vi "DAC Configure.vi"(8 "error in":errorcluster, 11 "DAC Vacum Pressure in":refnum<class "DAC Vacum Pressure.lvclass">) -> (0 "error out":errorcluster, 3 "DAC Vacum Pressure out":refnum<class "DAC Vacum Pressure.lvclass">)   [LabVIEW 2019, in "DAC.lvlib" / "DAC Vacum Pressure.lvclass"]
uses:
  DAC Vacum Pressure.lvclass
  C:/Users/krio/Documents/LV_Projects/test-stand/App/DAC/DAC.lvclass
  DAC.lvclass/DAC.ctl
  DAC Vacum Pressure.lvclass/DAC Vacum Pressure.ctl
  DAC.lvclass
  <vilib>/DAQmx/create/channels.llb/DAQmx Create Channel (AI-Current-Basic).vi
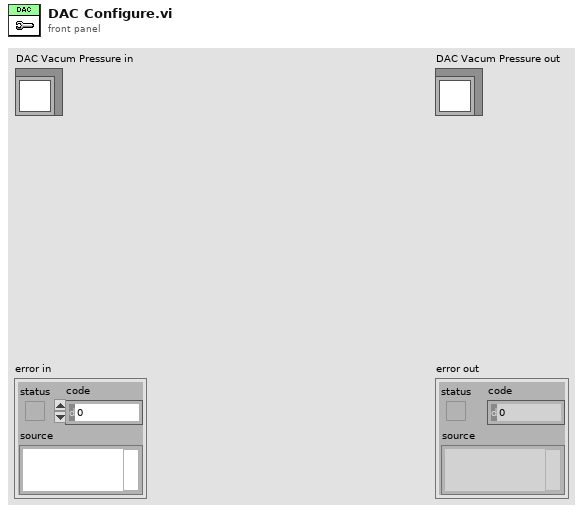
[diagram p1: front panel]
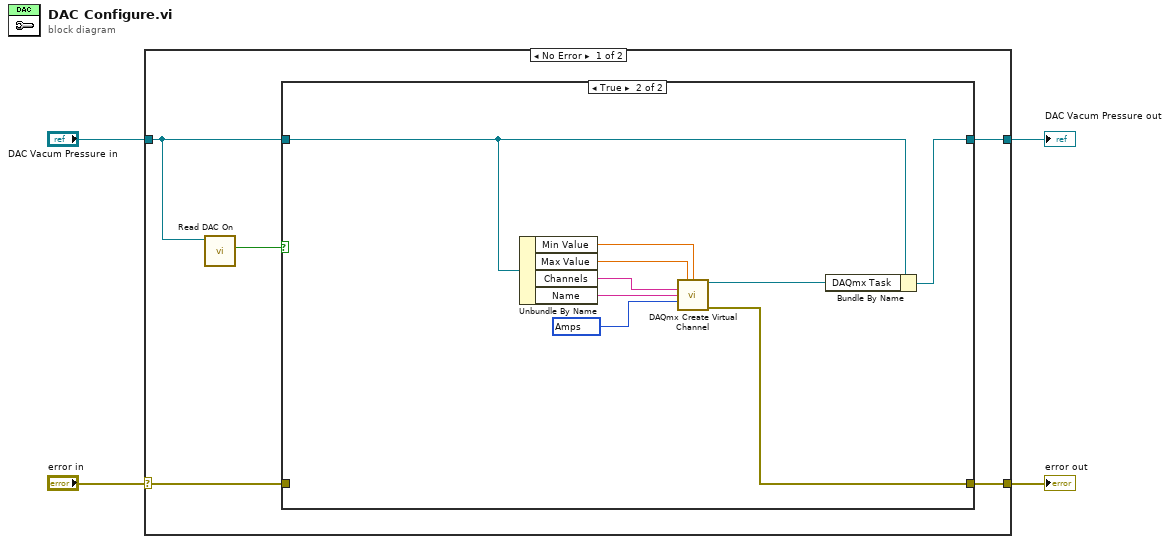
[diagram p0: block diagram]
diagram:
  n1 = case shown="No Error" "error in" {
    selector: "error in" -> [w6 w22]
    tunnel: [w5 w22] -> w4
    tunnel: [w7 w21] -> w3
    tunnel: "DAC Vacum Pressure in" -> [w9 w21]
    frame No Error {
      n2 = call "Read DAC On.vi"("DAC in"=w9) -> ("DAC On"=w8:bool)  [unwired: 8 in, 2 out]
      n3 = case shown="True" w8 {
        tunnel: w9 -> [w11 w19]
        tunnel: [w11 w18] -> w7
        tunnel: w6 -> [w10 _]
        tunnel: [w10 w16] -> w5
        frame False {
          # "Temperature measurement is off."
        }
        frame True {
          w12 = 10342 items=["Amps"=10342, "From Custom Scale"=10065] ("units")
          # "Temperature measurement is on."
          n4 = Unbundle By Name(w19) -> ("Min Value"=w13:dbl, "Max Value"=w20:dbl, "Channels"=w15:string, "Name"=w14:string)
          n5 = call-poly <vilib>:"DAQmx Create Virtual Channel.vi"("maximum value"=w20, "minimum value"=w13, "physical channels"=w15, "name to assign"=w14, "units"=w12) -> ("task out"=w17:refnum<k21>, "error out"=w16:errorcluster)  [unwired: 9 in]
          n6 = Bundle By Name(cluster=w19, "DAQmx Task"=w17) -> (w18:refnum<class "DAC Vacum Pressure.lvclass">)
        }
      }
    }
    frame Error {
    }
  }
  "error out" <- w4
  "DAC Vacum Pressure out" <- w3
